vi "Tower_Crane_Jack_Monitor.vi"() -> ()   [LabVIEW 2018]
uses:
  <vilib>/Utility/error.llb/DialogType.ctl
panel:
  out "起升高度（m）":dbl caption="起升高度（cm）" format="%#_3g"
  out "变幅长度（m）":dbl format="%#_3g"
  out "风速（m/s）":dbl format="%.3f"
  out "Y倾斜角度":dbl format="%#_3g"
  out "X倾斜角度":dbl format="%#_3g"
  out "回转角度（°）":dbl format="%#_3g"
  out "回转角度":dbl(knob) scale=0.0..10.0
  out "风速":dbl(knob) scale=0.0..10.0
  out "变幅长度":dbl(knob) scale=0.0..140.0
  out "y轴倾角":dbl(knob) scale=0.0..5.0
  out "x轴倾角":dbl(knob) scale=0.0..5.0
  out "温度计":dbl(slide) caption="顶升高度          (cm)" scale=0.0..180.0
  out "section_connect":picture caption="引进节连接"
  out "rotary_support":picture caption="下回转支座"
  out "stanard_section":picture caption="引进节"
  out "pin_shaft":picture caption="爬爪"
  out "jacking_beam":picture caption="顶升横梁"
  out "new picture":picture caption="Opertion_Guide"
  out "引进滑轮":bool
  out "引进节螺栓4":bool
  out "引进节螺栓3":bool
  out "引进节螺栓2":bool
  out "引进节螺栓1":bool
  out "下回转螺栓4":bool
  out "下回转螺栓3":bool
  out "下回转螺栓2":bool
  out "下回转螺栓1":bool
  out "爬爪右侧":bool
  out "爬爪左侧":bool
  out "横梁右侧":bool
  out "横梁左侧":bool
  in  "停止":bool
  in  "倾角串口号":refnum<visa-resource-name>
  in  "风速串口号":refnum<visa-resource-name>
  in  "回转编码器":refnum<visa-resource-name>
  in  "变幅编码器":refnum<visa-resource-name>
  in  "高度编码器":refnum<visa-resource-name>
  in  "顶升开关":bool
  in  "滚轮直径D":dbl
  out "esp32的IP地址":string
  out "回转圈数":dbl
  out "回转编码器读取缓冲区":string
  out "回转单圈值":dbl
  out "回转编码器错误输出":string
  out "变幅圈数":dbl
  out "小车蝙蝠编码器读取缓冲区":string
  out "变幅单圈值":dbl
  out "回转编码器错误输出1":string
  out "倾角读取缓冲区":string
  out "Wind_Speed_Data":string
  out "风速传感器错误输出":string
  out "操作规范":string
  out "起升圈数":dbl
  out "起升高度编码器读取缓冲区 2":string
  out "起升单圈值":dbl
  out "起升高度编码器数值":dbl
  out "高度编码器错误输出1":string
  out "data out":string
  out "数据输出":string
  out "信息来源的端口":u16
  in  "清空":bool
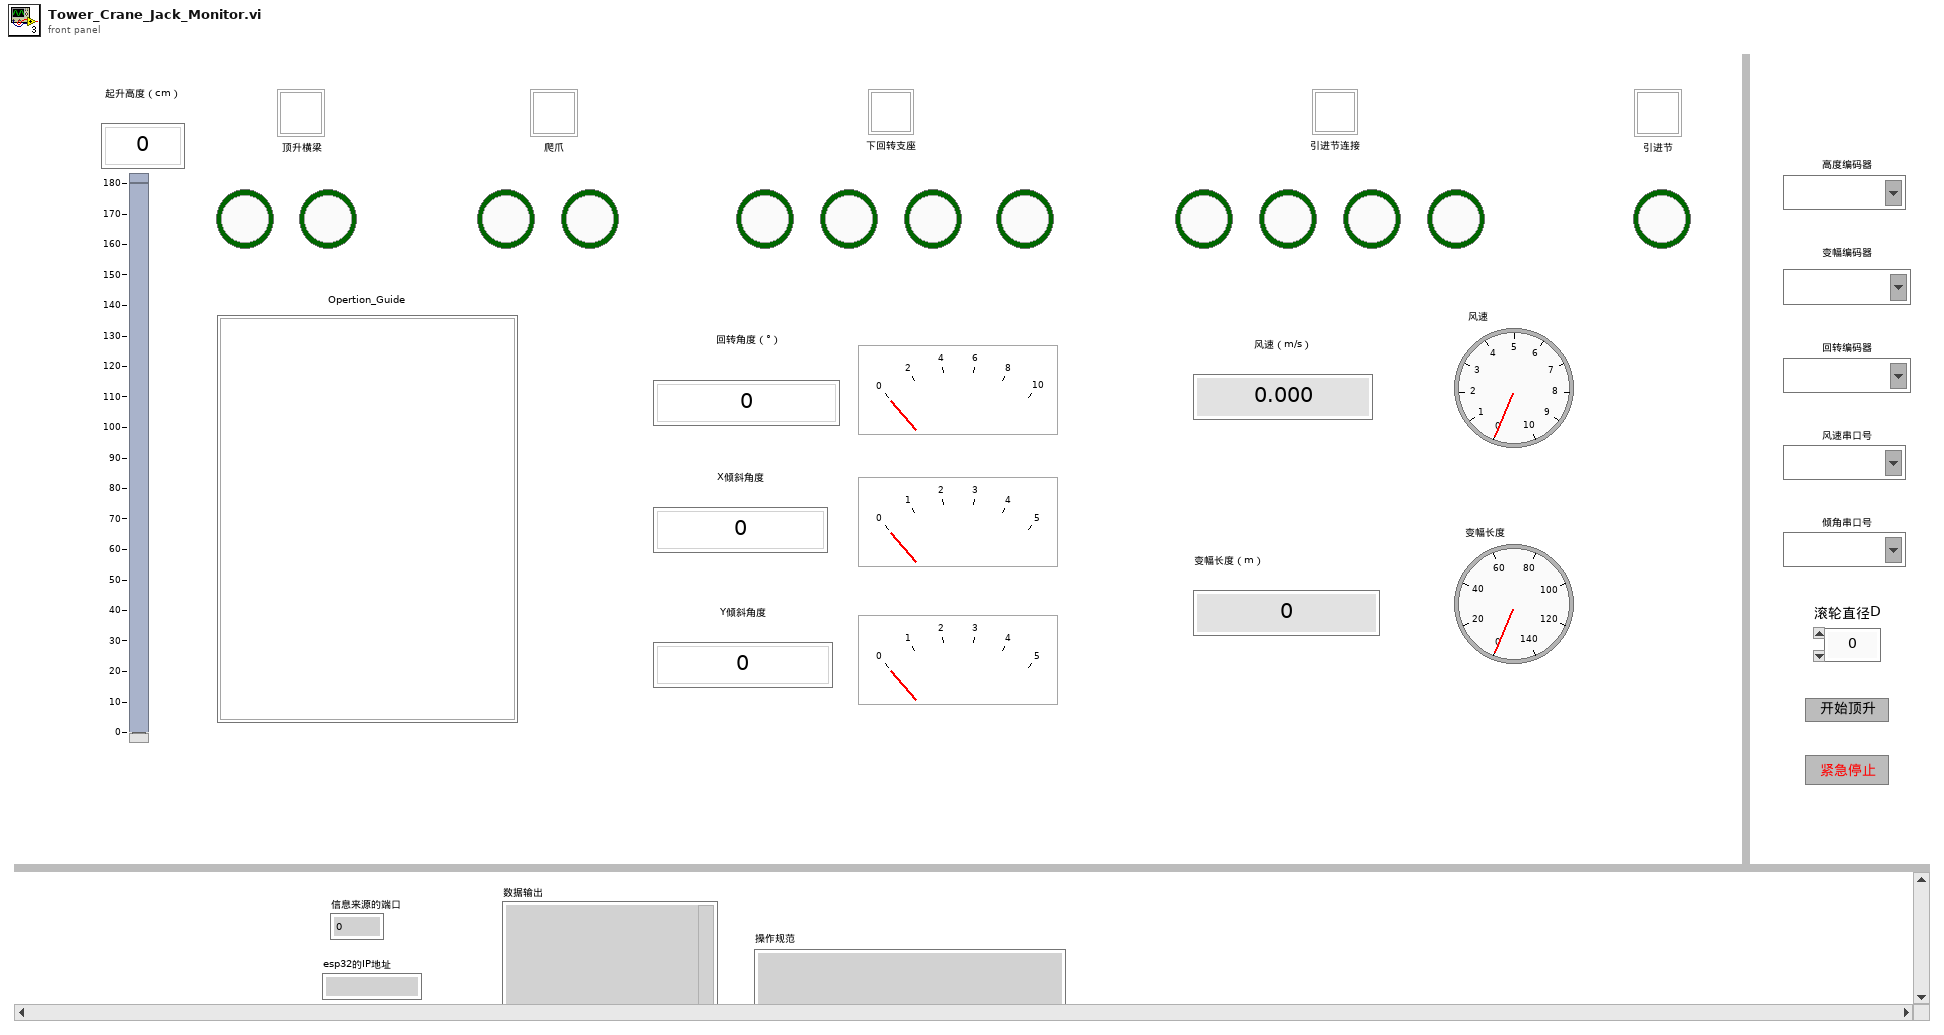
[diagram p1: front panel]
types:
  T1 = typedef "DialogType.ctl" = u16
  T2 = typedef "imagedata.ctl" = cluster{"image type":i32, "image depth":i32, "image":u8[], "mask":u8[], "colors":u32[], "Rectangle":cluster{"left":i16, "top":i16, "right":i16, "bottom":i16}}
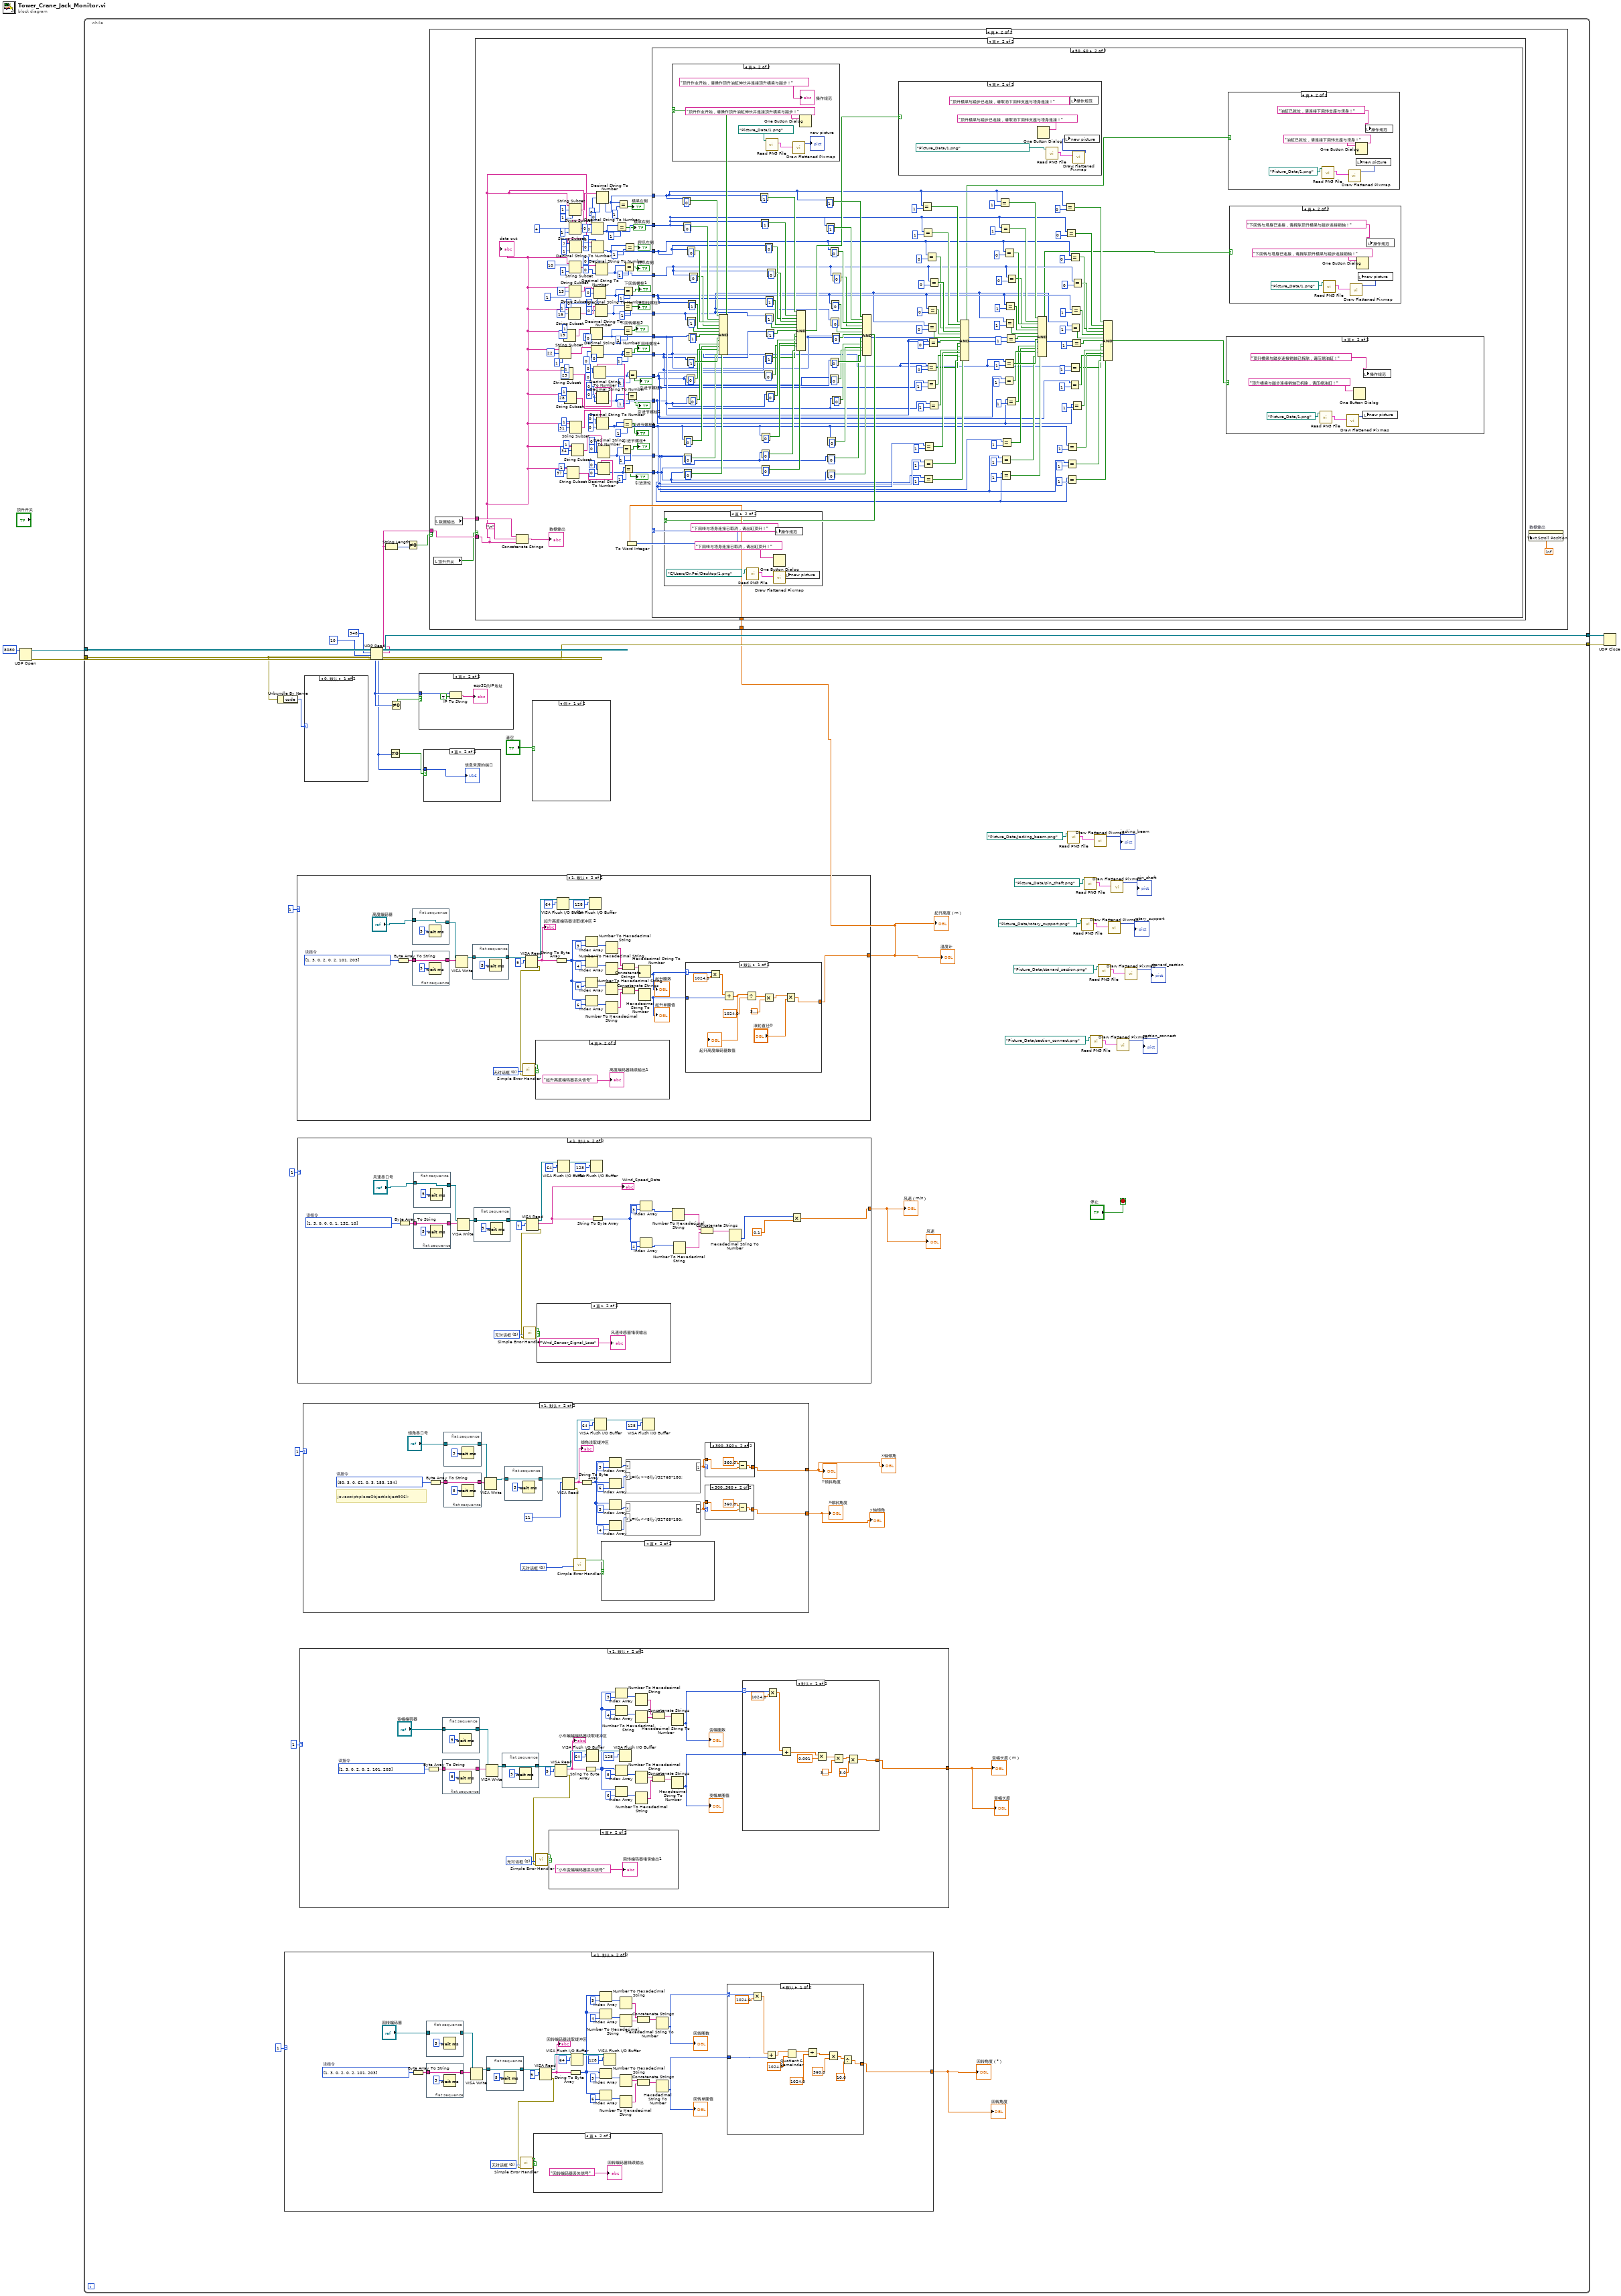
[diagram p0: block diagram]
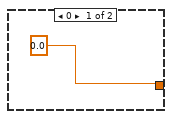
[diagram p2: hidden frame]
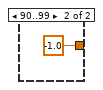
[diagram p4: hidden frame]
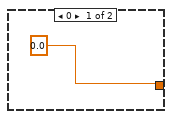
[diagram p5: hidden frame]
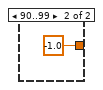
[diagram p7: hidden frame]
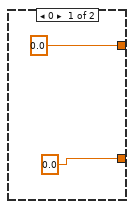
[diagram p8: hidden frame]
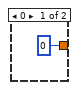
[diagram p12: hidden frame]
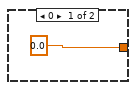
[diagram p14: hidden frame]
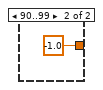
[diagram p16: hidden frame]
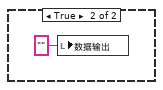
[diagram p17: hidden frame]
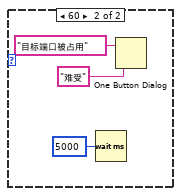
[diagram p18: hidden frame]
diagram:
  n1 = UDP Open(11:u16 8080 ("端口")) -> (port=w5:refnum<k16>, 0:w4:errorcluster)  [unwired: 4 in, 1 out]
  n2 = while {
    tunnel: w5 -> [w47]
    tunnel: w4 -> [w36]
    tunnel: [w46] -> w3
    tunnel: [w43] -> w2
    stop <- "停止" stop-if-true
    n3 = Unbundle By Name(w36) -> ("code"=w35:i32)
    n4 = case shown="1, 默认" 1 {
      tunnel: [0.0 w54] -> w6
      frame 0 {
      }
      frame 1, Default {
        w52 = T1 0 items=["无对话框", "确定信息", "继续或停止信息", "确定信息＋警告", "继续/停止+警告"] ("type of dialog (OK msg:1)")
        w55 = i32[] [1, 3, 0, 2, 0, 2, 101, 203]  # 读指令
        n5 = Byte Array To String(unsigned byte array=w55) -> (string=w72:string)
        n6 = flat-sequence {
          tunnel: "回转编码器" -> [w102]
          tunnel: [w102] -> w49
          frame #0 {
            n7 = Wait (ms)(milliseconds to wait=5) -> ()  [unwired: 1 out]
          }
        }
        n8 = flat-sequence {
          tunnel: [w100] -> w71
          tunnel: w72 -> [w100]
          frame #0 {
            n9 = Wait (ms)(milliseconds to wait=5) -> ()  [unwired: 1 out]
          }
        }
        n10 = VISA Write(VISA resource name=w49, write buffer=w71) -> (VISA resource name out=w63:refnum<visa-resource-name>)  [unwired: 1 in, 2 out]
        n11 = flat-sequence {
          tunnel: [w98] -> w64
          tunnel: w63 -> [w98]
          frame #0 {
            n12 = Wait (ms)(milliseconds to wait=5) -> ()  [unwired: 1 out]
          }
        }
        n13 = VISA Read(VISA resource name=w64, byte count=u32 9 ("字节总数")) -> (VISA resource name out=w80:refnum<visa-resource-name>, read buffer=w70:string, error out=w51:errorcluster)  [unwired: 1 in, 1 out]
        "回转编码器读取缓冲区" <- w70
        n14 = call <vilib>:"Simple Error Handler.vi"("type of dialog (OK msg:1)"=w52, "error in (no error)"=w51) -> ("error?"=w53:bool)  [unwired: 3 in, 4 out]
        n15 = case shown="真" w53 {
          frame False {
          }
          frame True {
            "回转编码器错误输出" <- "回转编码器丢失信号" ("九轴错误输出1")
          }
        }
        n16 = String To Byte Array(string=w70) -> (unsigned byte array=w78:u8[])
        n17 = VISA Flush I/O Buffer(VISA resource name=w80, mask (16)=64) -> (VISA resource name out=w79:refnum<visa-resource-name>)  [unwired: 1 in, 1 out]
        n18 = Index Array ("索引数组")(array=w78, index=3) -> (element=w65:u8)
        n19 = Index Array(array=w78, index=4) -> (element=w69:u8)
        n20 = Index Array ("索引数组")(array=w78, index=5) -> (element=w73:u8)
        n21 = Index Array(array=w78, index=6) -> (element=w77:u8)
        n22 = VISA Flush I/O Buffer(VISA resource name=w79, mask (16)=128) -> ()  [unwired: 1 in, 2 out]
        n23 = Number To Hexadecimal String(2:w65) -> (0:w68:string)  [unwired: 1 in]
        n24 = Number To Hexadecimal String(2:w69) -> (0:w67:string)  [unwired: 1 in]
        n25 = Number To Hexadecimal String(2:w73) -> (0:w76:string)  [unwired: 1 in]
        n26 = Number To Hexadecimal String(2:w77) -> (0:w75:string)  [unwired: 1 in]
        n27 = Concatenate Strings(w68, w67) -> (w66:string)
        n28 = Concatenate Strings(w76, w75) -> (w74:string)
        n29 = Hexadecimal String To Number(string=w66) -> (number=w81:u32)  [unwired: 2 in, 1 out]
        "回转圈数" <- w81
        n30 = Hexadecimal String To Number(string=w74) -> (number=w82:u32)  [unwired: 2 in, 1 out]
        "回转单圈值" <- w82
        n31 = case shown="默认" w81 {
          selector: w81 -> [w94 _]
          tunnel: w82 -> [w93 _]
          tunnel: [w85 -1.0] -> w54
          frame Default {
            n32 = Multiply(x=w94, y=1024.0) -> (x*y=w96:dbl)
            n33 = Add(x=w96, y=w93) -> (x+y=w92:dbl)
            n34 = Quotient & Remainder(x=w92, y=1024.0) -> (x-y*floor(x/y)=w87:dbl)  [unwired: 1 out]
            n35 = Divide(x=w87, y=1024.0) -> (x/y=w89:dbl)
            n36 = Multiply(x=w89, y=360.0) -> (x*y=w86:dbl)
            n37 = Divide(x=w86, y=10.0) -> (x/y=w85:dbl)
          }
          frame 90..99 {
          }
        }
      }
    }
    "回转角度（°）" <- w6
    "回转角度" <- w6
    n38 = case shown="1, 默认" 1 {
      tunnel: [0.0 w244] -> w11
      frame 0 {
      }
      frame 1, Default {
        w242 = T1 0 items=["无对话框", "确定信息", "继续或停止信息", "确定信息＋警告", "继续/停止+警告"] ("type of dialog (OK msg:1)")
        w245 = i32[] [1, 3, 0, 2, 0, 2, 101, 203]  # 读指令
        n39 = Byte Array To String(unsigned byte array=w245) -> (string=w261:string)
        n40 = flat-sequence {
          tunnel: "高度编码器" -> [w290]
          tunnel: [w290] -> w239
          frame #0 {
            n41 = Wait (ms)(milliseconds to wait=5) -> ()  [unwired: 1 out]
          }
        }
        n42 = flat-sequence {
          tunnel: [w288] -> w260
          tunnel: w261 -> [w288]
          frame #0 {
            n43 = Wait (ms)(milliseconds to wait=5) -> ()  [unwired: 1 out]
          }
        }
        n44 = VISA Write(VISA resource name=w239, write buffer=w260) -> (VISA resource name out=w253:refnum<visa-resource-name>)  [unwired: 1 in, 2 out]
        n45 = flat-sequence {
          tunnel: [w286] -> w254
          tunnel: w253 -> [w286]
          frame #0 {
            n46 = Wait (ms)(milliseconds to wait=5) -> ()  [unwired: 1 out]
          }
        }
        n47 = VISA Read(VISA resource name=w254, byte count=u32 9 ("字节总数")) -> (VISA resource name out=w269:refnum<visa-resource-name>, read buffer=w270:string, error out=w241:errorcluster)  [unwired: 1 in, 1 out]
        "起升高度编码器读取缓冲区 2" <- w270
        n48 = call <vilib>:"Simple Error Handler.vi"("type of dialog (OK msg:1)"=w242, "error in (no error)"=w241) -> ("error?"=w243:bool)  [unwired: 3 in, 4 out]
        n49 = case shown="真" w243 {
          frame False {
          }
          frame True {
            "高度编码器错误输出1" <- "起升高度编码器丢失信号" ("九轴错误输出1")
          }
        }
        n50 = String To Byte Array(string=w270) -> (unsigned byte array=w267:u8[])
        n51 = VISA Flush I/O Buffer(VISA resource name=w269, mask (16)=64) -> (VISA resource name out=w268:refnum<visa-resource-name>)  [unwired: 1 in, 1 out]
        n52 = Index Array ("索引数组")(array=w267, index=3) -> (element=w255:u8)
        n53 = Index Array(array=w267, index=4) -> (element=w259:u8)
        n54 = Index Array ("索引数组")(array=w267, index=5) -> (element=w262:u8)
        n55 = Index Array(array=w267, index=6) -> (element=w266:u8)
        n56 = VISA Flush I/O Buffer(VISA resource name=w268, mask (16)=128) -> ()  [unwired: 1 in, 2 out]
        n57 = Number To Hexadecimal String(2:w255) -> (0:w258:string)  [unwired: 1 in]
        n58 = Number To Hexadecimal String(2:w259) -> (0:w257:string)  [unwired: 1 in]
        n59 = Number To Hexadecimal String(2:w262) -> (0:w265:string)  [unwired: 1 in]
        n60 = Number To Hexadecimal String(2:w266) -> (0:w264:string)  [unwired: 1 in]
        n61 = Concatenate Strings(w258, w257) -> (w256:string)
        n62 = Concatenate Strings(w265, w264) -> (w263:string)
        n63 = Hexadecimal String To Number(string=w256) -> (number=w271:u32)  [unwired: 2 in, 1 out]
        "起升圈数" <- w271
        n64 = Hexadecimal String To Number(string=w263) -> (number=w272:u32)  [unwired: 2 in, 1 out]
        "起升单圈值" <- w272
        n65 = case shown="默认" w271 {
          selector: w271 -> [w281 _]
          tunnel: w272 -> [w282 _]
          tunnel: [w274 -1.0] -> w244
          frame Default {
            n66 = Multiply(x=w281, y=1024.0) -> (x*y=w284:dbl)
            n67 = Add(x=w284, y=w282) -> (x+y=w280:dbl)
            "起升高度编码器数值" <- w280
            n68 = Divide(x=w280, y=1024.0) -> (x/y=w278:dbl)
            n69 = Multiply(x=w278, y=3.141592653589793) -> (x*y=w276:dbl)
            n70 = Multiply(x=w276, y="滚轮直径D") -> (x*y=w274:dbl)
          }
          frame 90..99 {
          }
        }
      }
    }
    "起升高度（m）" <- w11
    "温度计" <- w11
    n71 = case shown="1, 默认" 1 {
      tunnel: [u32 0 w205] -> w7
      frame 0 {
      }
      frame 1, Default {
        w219 = T1 0 items=["无对话框", "确定信息", "继续或停止信息", "确定信息＋警告", "继续/停止+警告"] ("type of dialog (OK msg:1)")
        w221 = i32[] [1, 3, 0, 0, 0, 1, 132, 10]  # 读指令
        n72 = Byte Array To String(unsigned byte array=w221) -> (string=w228:string)
        n73 = flat-sequence {
          tunnel: "风速串口号" -> [w236]
          tunnel: [w236] -> w216
          frame #0 {
            n74 = Wait (ms)(milliseconds to wait=5) -> ()  [unwired: 1 out]
          }
        }
        n75 = flat-sequence {
          tunnel: [w234] -> w227
          tunnel: w228 -> [w234]
          frame #0 {
            n76 = Wait (ms)(milliseconds to wait=5) -> ()  [unwired: 1 out]
          }
        }
        n77 = VISA Write(VISA resource name=w216, write buffer=w227) -> (VISA resource name out=w225:refnum<visa-resource-name>)  [unwired: 1 in, 2 out]
        n78 = flat-sequence {
          tunnel: [w232] -> w226
          tunnel: w225 -> [w232]
          frame #0 {
            n79 = Wait (ms)(milliseconds to wait=5) -> ()  [unwired: 1 out]
          }
        }
        n80 = VISA Read(VISA resource name=w226, byte count=u32 7 ("字节总数")) -> (VISA resource name out=w230:refnum<visa-resource-name>, read buffer=w215:string, error out=w218:errorcluster)  [unwired: 1 in, 1 out]
        "Wind_Speed_Data" <- w215
        n81 = call <vilib>:"Simple Error Handler.vi"("type of dialog (OK msg:1)"=w219, "error in (no error)"=w218) -> ("error?"=w220:bool)  [unwired: 3 in, 4 out]
        n82 = case shown="真" w220 {
          frame False {
          }
          frame True {
            "风速传感器错误输出" <- "Wnd_Sensor_Signal_Loss" ("九轴错误输出1")
          }
        }
        n83 = VISA Flush I/O Buffer(VISA resource name=w230, mask (16)=64) -> (VISA resource name out=w229:refnum<visa-resource-name>)  [unwired: 1 in, 1 out]
        n84 = VISA Flush I/O Buffer(VISA resource name=w229, mask (16)=128) -> ()  [unwired: 1 in, 2 out]
        n85 = String To Byte Array(string=w215) -> (unsigned byte array=w214:u8[])
        n86 = Index Array(array=w214, index=3 ("索引")) -> (element=w211:u8)
        n87 = Index Array(array=w214, index=4 ("索引")) -> (element=w210:u8)
        n88 = Number To Hexadecimal String(2:w211) -> (0:w209:string)  [unwired: 1 in]
        n89 = Number To Hexadecimal String(2:w210) -> (0:w208:string)  [unwired: 1 in]
        n90 = Concatenate Strings(w209, w208) -> (w207:string)
        n91 = Hexadecimal String To Number(string=w207) -> (number=w206:u32)  [unwired: 2 in, 1 out]
        n92 = Multiply(x=w206, y=0.1) -> (x*y=w205:dbl)
      }
    }
    "风速" <- w7
    "风速（m/s）" <- w7
    n93 = case shown="1, 默认" 1 {
      tunnel: [0.0 w110] -> w8
      frame 0 {
      }
      frame 1, Default {
        w108 = T1 0 items=["无对话框", "确定信息", "继续或停止信息", "确定信息＋警告", "继续/停止+警告"] ("type of dialog (OK msg:1)")
        w111 = i32[] [1, 3, 0, 2, 0, 2, 101, 203]  # 读指令
        n94 = Byte Array To String(unsigned byte array=w111) -> (string=w128:string)
        n95 = flat-sequence {
          tunnel: "变幅编码器" -> [w156]
          tunnel: [w156] -> w105
          frame #0 {
            n96 = Wait (ms)(milliseconds to wait=5) -> ()  [unwired: 1 out]
          }
        }
        n97 = flat-sequence {
          tunnel: [w154] -> w127
          tunnel: w128 -> [w154]
          frame #0 {
            n98 = Wait (ms)(milliseconds to wait=5) -> ()  [unwired: 1 out]
          }
        }
        n99 = VISA Write(VISA resource name=w105, write buffer=w127) -> (VISA resource name out=w119:refnum<visa-resource-name>)  [unwired: 1 in, 2 out]
        n100 = flat-sequence {
          tunnel: [w152] -> w120
          tunnel: w119 -> [w152]
          frame #0 {
            n101 = Wait (ms)(milliseconds to wait=5) -> ()  [unwired: 1 out]
          }
        }
        n102 = VISA Read(VISA resource name=w120, byte count=u32 9 ("字节总数")) -> (VISA resource name out=w136:refnum<visa-resource-name>, read buffer=w126:string, error out=w107:errorcluster)  [unwired: 1 in, 1 out]
        "小车蝙蝠编码器读取缓冲区" <- w126
        n103 = call <vilib>:"Simple Error Handler.vi"("type of dialog (OK msg:1)"=w108, "error in (no error)"=w107) -> ("error?"=w109:bool)  [unwired: 3 in, 4 out]
        n104 = case shown="真" w109 {
          frame False {
          }
          frame True {
            "回转编码器错误输出1" <- "小车变幅编码器丢失信号" ("九轴错误输出1")
          }
        }
        n105 = String To Byte Array(string=w126) -> (unsigned byte array=w134:u8[])
        n106 = VISA Flush I/O Buffer(VISA resource name=w136, mask (16)=64) -> (VISA resource name out=w135:refnum<visa-resource-name>)  [unwired: 1 in, 1 out]
        n107 = Index Array ("索引数组")(array=w134, index=3) -> (element=w121:u8)
        n108 = Index Array(array=w134, index=4) -> (element=w125:u8)
        n109 = Index Array ("索引数组")(array=w134, index=5) -> (element=w129:u8)
        n110 = Index Array(array=w134, index=6) -> (element=w133:u8)
        n111 = VISA Flush I/O Buffer(VISA resource name=w135, mask (16)=128) -> ()  [unwired: 1 in, 2 out]
        n112 = Number To Hexadecimal String(2:w121) -> (0:w124:string)  [unwired: 1 in]
        n113 = Number To Hexadecimal String(2:w125) -> (0:w123:string)  [unwired: 1 in]
        n114 = Number To Hexadecimal String(2:w129) -> (0:w132:string)  [unwired: 1 in]
        n115 = Number To Hexadecimal String(2:w133) -> (0:w131:string)  [unwired: 1 in]
        n116 = Concatenate Strings(w124, w123) -> (w122:string)
        n117 = Concatenate Strings(w132, w131) -> (w130:string)
        n118 = Hexadecimal String To Number(string=w122) -> (number=w137:u32)  [unwired: 2 in, 1 out]
        "变幅圈数" <- w137
        n119 = Hexadecimal String To Number(string=w130) -> (number=w138:u32)  [unwired: 2 in, 1 out]
        "变幅单圈值" <- w138
        n120 = case shown="默认" w137 {
          selector: w137 -> [w144 _]
          tunnel: w138 -> [w143 _]
          tunnel: [w142 -1.0] -> w110
          frame Default {
            n121 = Multiply(x=w144, y=1024.0) -> (x*y=w149:dbl)
            n122 = Add(x=w149, y=w143) -> (x+y=w150:dbl)
            n123 = Multiply(x=w150, y=0.001) -> (x*y=w147:dbl)
            n124 = Multiply(x=w147, y=3.141592653589793) -> (x*y=w148:dbl)
            n125 = Multiply(x=w148, y=3.0) -> (x*y=w142:dbl)
          }
          frame 90..99 {
          }
        }
      }
    }
    "变幅长度（m）" <- w8
    "变幅长度" <- w8
    n126 = case shown="1, 默认" 1 {
      tunnel: [0.0 w166] -> w10
      tunnel: [0.0 w165] -> w9
      frame 0 {
      }
      frame 1, Default {
        w162 = T1 0 items=["无对话框", "确定信息", "继续或停止信息", "确定信息＋警告", "继续/停止+警告"] ("type of dialog (OK msg:1)")
        w167 = i32[] [80, 3, 0, 61, 0, 3, 153, 134]  # 读指令
        # "javascript:placeObject(object906);"
        n127 = Byte Array To String(unsigned byte array=w167) -> (string=w180:string)
        n128 = flat-sequence {
          tunnel: [w201] -> w161
          tunnel: "倾角串口号" -> [w201]
          frame #0 {
            n129 = Wait (ms)(milliseconds to wait=5) -> ()  [unwired: 1 out]
          }
        }
        n130 = flat-sequence {
          tunnel: [w199] -> w181
          tunnel: w180 -> [w199]
          frame #0 {
            n131 = Wait (ms)(milliseconds to wait=5) -> ()  [unwired: 1 out]
          }
        }
        n132 = VISA Write(VISA resource name=w161, write buffer=w181) -> (VISA resource name out=w176:refnum<visa-resource-name>)  [unwired: 1 in, 2 out]
        n133 = flat-sequence {
          tunnel: w176 -> [w197]
          tunnel: [w197] -> w177
          frame #0 {
            n134 = Wait (ms)(milliseconds to wait=5) -> ()  [unwired: 1 out]
          }
        }
        n135 = VISA Read(VISA resource name=w177, byte count=u32 11 ("字节总数")) -> (VISA resource name out=w185:refnum<visa-resource-name>, read buffer=w175:string, error out=w163:errorcluster)  [unwired: 1 in, 1 out]
        "倾角读取缓冲区" <- w175
        n136 = call <vilib>:"Simple Error Handler.vi"("type of dialog (OK msg:1)"=w162, "error in (no error)"=w163) -> ("error?"=w164:bool)  [unwired: 3 in, 4 out]
        n137 = String To Byte Array(string=w175) -> (unsigned byte array=w186:u8[])
        n138 = VISA Flush I/O Buffer(VISA resource name=w185, mask (16)=64) -> (VISA resource name out=w184:refnum<visa-resource-name>)  [unwired: 1 in, 1 out]
        n139 = case shown="真" w164 {
          frame False {
          }
          frame True {
          }
        }
        n140 = Index Array(array=w186, index=5) -> (element=w183:u8)
        n141 = Index Array(array=w186, index=6) -> (element=w182:u8)
        n142 = Index Array(array=w186, index=3) -> (element=w179:u8)
        n143 = Index Array(array=w186, index=4) -> (element=w178:u8)
        n144 = formula code="z=((x<<8)|y)/32768*180;"("x"=w183, "y"=w182) -> ("z"=w188:dbl)
        n145 = formula code="z=((x<<8)|y)/32768*180;"("x"=w179, "y"=w178) -> ("z"=w187:dbl)
        n146 = VISA Flush I/O Buffer(VISA resource name=w184, mask (16)=128) -> ()  [unwired: 1 in, 2 out]
        n147 = case shown="300..360" w188 {
          tunnel: [w193 w195] -> w166
          tunnel: w188 -> [w193 w194]
          frame Default {
          }
          frame 300..360 {
            n148 = Subtract(x=360.0, y=w194) -> (x-y=w195:dbl)
          }
        }
        n149 = case shown="300..360" w187 {
          tunnel: [w189 w191] -> w165
          tunnel: w187 -> [w189 w190]
          frame Default {
          }
          frame 300..360 {
            n150 = Subtract(x=360.0, y=w190) -> (x-y=w191:dbl)
          }
        }
      }
    }
    "X倾斜角度" <- w9
    "Y倾斜角度" <- w10
    "x轴倾角" <- w10
    "y轴倾角" <- w9
    n151 = case shown="0, 默认" w35 {
      frame 0, Default {
      }
      frame 60 {
        n152 = Wait (ms)(milliseconds to wait=u32 5000 ("等待时间（毫秒）")) -> ()  [unwired: 1 out]
        n153 = One Button Dialog(message="目标端口被占用" ("消息"), button name ("OK")="难受" ("按钮名称（“确定”）")) -> ()  [unwired: 1 out]
      }
    }
    n154 = UDP Read(connection ID=w47, max size (548)=548 ("最大值(548)"), timeout ms (25000)=10 ("超时毫秒(25000)"), 8:w36) -> (data out=w40:string, error out=w46:errorcluster, 3:w43:refnum<k16>, 4:w34:u16, 6:w39:u32)
    n155 = String Length(string=w40) -> (length=w42:i32)
    n156 = Not Equal To 0?(x=w34) -> (x != 0?=w37:bool)
    n157 = Not Equal To 0?(x=w39) -> (x != 0?=w38:bool)
    n158 = Not Equal To 0?(x=w42) -> (x != 0?=w41:bool)
    n159 = case shown="真" w38 {
      tunnel: w39 -> [_ w299]
      frame False {
      }
      frame True {
        n160 = IP To String(1:TRUE ("句点符号？(F)"), 2:w299) -> (0:→"esp32的IP地址":string)
      }
    }
    n161 = case shown="真" w37 {
      tunnel: w34 -> [_ w296]
      frame False {
      }
      frame True {
        "信息来源的端口" <- w296
      }
    }
    n162 = case shown="真" w41 {
      tunnel: w40 -> [_ w303]
      tunnel: w11 -> [_ w301]
      frame False {
      }
      frame True {
        n163 = local read "顶升开关"() -> (w300:bool)
        n164 = local read "数据输出"() -> (w304:string)
        n165 = case shown="真" w300 {
          tunnel: w304 -> [w307 w416]
          tunnel: w303 -> [w306 w391]
          tunnel: w301 -> [_ w394]
          frame False {
            n166 = Concatenate Strings(w307, w306) -> (w305:string)
            n167 = local write "数据输出"(w305) -> ()
          }
          frame True {
            (unwired) 0 ("默认(0 I32)")
            n168 = Concatenate Strings(w416, "\n", w391) -> (→"数据输出":string)
            n169 = String Subset(string=w391, offset (0)=22 ("偏移量(0)"), length (rest)=1 ("长度（剩余）")) -> (substring=w352:string)
            n170 = String Subset(string=w391, offset (0)=25 ("偏移量(0)"), length (rest)=1 ("长度（剩余）")) -> (substring=w351:string)
            n171 = String Subset(string=w391, offset (0)=19 ("偏移量(0)"), length (rest)=1 ("长度（剩余）")) -> (substring=w353:string)
            n172 = String Subset(string=w391, offset (0)=28 ("偏移量(0)"), length (rest)=1 ("长度（剩余）")) -> (substring=w350:string)
            n173 = String Subset(string=w391, offset (0)=37 ("偏移量(0)"), length (rest)=1 ("长度（剩余）")) -> (substring=w347:string)
            n174 = String Subset(string=w391, offset (0)=16 ("偏移量(0)"), length (rest)=1 ("长度（剩余）")) -> (substring=w369:string)
            n175 = String Subset(string=w391, offset (0)=4 ("偏移量(0)"), length (rest)=1 ("长度（剩余）")) -> (substring=w404:string)
            n176 = String Subset(string=w391, offset (0)=13 ("偏移量(0)"), length (rest)=1 ("长度（剩余）")) -> (substring=w370:string)
            n177 = String Subset(string=w391, offset (0)=1 ("偏移量(0)"), length (rest)=1 ("长度（剩余）")) -> (substring=w406:string)
            n178 = String Subset(string=w391, offset (0)=10 ("偏移量(0)"), length (rest)=1 ("长度（剩余）")) -> (substring=w403:string)
            n179 = String Subset(string=w391, offset (0)=31 ("偏移量(0)"), length (rest)=1 ("长度（剩余）")) -> (substring=w349:string)
            n180 = String Subset(string=w391, offset (0)=7 ("偏移量(0)"), length (rest)=1 ("长度（剩余）")) -> (substring=w405:string)
            n181 = String Subset(string=w391, offset (0)=34 ("偏移量(0)"), length (rest)=1 ("长度（剩余）")) -> (substring=w348:string)
            n182 = Decimal String To Number(string=w353, offset=0 ("偏移量"), default (0L)=0 ("默认(0 I32)")) -> (number=w323:i32)  [unwired: 1 out]
            n183 = Decimal String To Number(string=w404, offset=0 ("偏移量"), default (0L)=0 ("默认(0 I32)")) -> (number=w331:i32)  [unwired: 1 out]
            n184 = Decimal String To Number(string=w352, offset=0 ("偏移量"), default (0L)=0 ("默认(0 I32)")) -> (number=w322:i32)  [unwired: 1 out]
            n185 = Decimal String To Number(string=w405, offset=0 ("偏移量"), default (0L)=0 ("默认(0 I32)")) -> (number=w329:i32)  [unwired: 1 out]
            n186 = Decimal String To Number(string=w370, offset=0 ("偏移量"), default (0L)=0 ("默认(0 I32)")) -> (number=w325:i32)  [unwired: 1 out]
            n187 = Decimal String To Number(string=w351, offset=0 ("偏移量")) -> (number=w321:i32)  [unwired: 1 in, 1 out]
            n188 = Decimal String To Number(string=w369, offset=0 ("偏移量"), default (0L)=0 ("默认(0 I32)")) -> (number=w324:i32)  [unwired: 1 out]
            n189 = Decimal String To Number(string=w403, offset=0 ("偏移量"), default (0L)=0 ("默认(0 I32)")) -> (number=w327:i32)  [unwired: 1 out]
            n190 = Decimal String To Number(string=w406, offset=0 ("偏移量"), default (0L)=0 ("默认(0 I32)")) -> (number=w346:i32)  [unwired: 1 out]
            n191 = Decimal String To Number(string=w350, offset=0 ("偏移量"), default (0L)=0 ("默认(0 I32)")) -> (number=w320:i32)  [unwired: 1 out]
            n192 = Decimal String To Number(string=w349, offset=0 ("偏移量"), default (0L)=0 ("默认(0 I32)")) -> (number=w319:i32)  [unwired: 1 out]
            n193 = Decimal String To Number(string=w348, offset=0 ("偏移量"), default (0L)=0 ("默认(0 I32)")) -> (number=w318:i32)  [unwired: 1 out]
            n194 = Decimal String To Number(string=w347, offset=0 ("偏移量"), default (0L)=0 ("默认(0 I32)")) -> (number=w317:i32)  [unwired: 1 out]
            n195 = Equal?(x=w331, y=1) -> (x = y?=→"横梁右侧":bool)
            n196 = Equal?(x=w346, y=1) -> (x = y?=→"横梁左侧":bool)
            n197 = Equal?(x=w318, y=1) -> (x = y?=→"引进节螺栓4":bool)
            n198 = Equal?(x=w319, y=1) -> (x = y?=→"引进节螺栓3":bool)
            n199 = Equal?(x=w324, y=1) -> (x = y?=→"下回转螺栓2":bool)
            n200 = Equal?(x=w323, y=1) -> (x = y?=→"下回转螺栓3":bool)
            n201 = Equal?(x=w322, y=1) -> (x = y?=→"下回转螺栓4":bool)
            n202 = Equal?(x=w325, y=1) -> (x = y?=→"下回转螺栓1":bool)
            n203 = Equal?(x=w317, y=1) -> (x = y?=→"引进滑轮":bool)
            n204 = Equal?(x=w327, y=1) -> (x = y?=→"爬爪右侧":bool)
            n205 = Equal?(x=w329, y=1) -> (x = y?=→"爬爪左侧":bool)
            n206 = To Word Integer(number=w394) -> (16bit integer=w393:i16)
            n207 = Equal?(x=w320, y=1) -> (x = y?=→"引进节螺栓2":bool)
            n208 = Equal?(x=w321, y=1) -> (x = y?=→"引进节螺栓1":bool)
            n209 = case shown="50..60" w393 {
              tunnel: w346 -> [w432 w547 w762 w840 w915 _ w997]
              tunnel: w331 -> [w431 w546 w763 w839 w914 _ w996]
              tunnel: w329 -> [w430 w545 w761 w838 w913 _ w995]
              tunnel: w327 -> [w429 w544 w760 w837 w912 _ w994]
              tunnel: w325 -> [w428 w543 w759 w836 w911 _ w993]
              tunnel: w324 -> [w427 w542 w758 w835 w910 _ w992]
              tunnel: w323 -> [w426 w541 w757 w834 w909 _ w991]
              tunnel: w322 -> [w425 w540 w756 w833 w908 _ w990]
              tunnel: w321 -> [w424 w539 w755 w832 w907 _ w989]
              tunnel: w320 -> [w423 w532 w754 w831 w906 _ w988]
              tunnel: w319 -> [w422 w538 w753 w830 w905 _ w987]
              tunnel: w318 -> [w421 w537 w752 w829 w904 _ w986]
              tunnel: w317 -> [w420 w536 w751 w828 w903 _ w985]
              frame 25..30, Default {
                n210 = Equal?(x=w432, y=0) -> (x = y?=w510:bool)
                n211 = Equal?(x=w431, y=0) -> (x = y?=w509:bool)
                n212 = Equal?(x=w421, y=0) -> (x = y?=w499:bool)
                n213 = Equal?(x=w420, y=0) -> (x = y?=w498:bool)
                n214 = Equal?(x=w422, y=0) -> (x = y?=w500:bool)
                n215 = Equal?(x=w424, y=0) -> (x = y?=w502:bool)
                n216 = Equal?(x=w430, y=1) -> (x = y?=w508:bool)
                n217 = Equal?(x=w425, y=0) -> (x = y?=w503:bool)
                n218 = Equal?(x=w427, y=0) -> (x = y?=w505:bool)
                n219 = Equal?(x=w428, y=0) -> (x = y?=w506:bool)
                n220 = Equal?(x=w426, y=0) -> (x = y?=w504:bool)
                n221 = Equal?(x=w423, y=0) -> (x = y?=w501:bool)
                n222 = Equal?(x=w429, y=1) -> (x = y?=w507:bool)
                n223 = Compound Arithmetic op=AND ("复合运算")(w510, w509, w508, w507, w506, w505, w504, w503, w502, w501, w500, w499, w498) -> (w419:bool)
                n224 = Equal?(x=w432, y=1) -> (x = y?=w485:bool)
                n225 = Equal?(x=w431, y=1) -> (x = y?=w486:bool)
                n226 = Equal?(x=w421, y=0) -> (x = y?=w496:bool)
                n227 = Equal?(x=w420, y=0) -> (x = y?=w497:bool)
                n228 = Equal?(x=w422, y=0) -> (x = y?=w495:bool)
                n229 = Equal?(x=w424, y=0) -> (x = y?=w493:bool)
                n230 = Equal?(x=w430, y=1) -> (x = y?=w487:bool)
                n231 = Equal?(x=w425, y=0) -> (x = y?=w492:bool)
                n232 = Equal?(x=w427, y=0) -> (x = y?=w490:bool)
                n233 = Equal?(x=w428, y=0) -> (x = y?=w489:bool)
                n234 = Equal?(x=w426, y=0) -> (x = y?=w491:bool)
                n235 = Equal?(x=w423, y=0) -> (x = y?=w494:bool)
                n236 = Equal?(x=w429, y=1) -> (x = y?=w488:bool)
                n237 = Compound Arithmetic op=AND ("复合运算")(w485, w486, w487, w488, w489, w490, w491, w492, w493, w494, w495, w496, w497) -> (w418:bool)
                n238 = Equal?(x=w432, y=1) -> (x = y?=w484:bool)
                n239 = Equal?(x=w431, y=1) -> (x = y?=w483:bool)
                n240 = Equal?(x=w421, y=0) -> (x = y?=w473:bool)
                n241 = Equal?(x=w420, y=0) -> (x = y?=w472:bool)
                n242 = Equal?(x=w422, y=0) -> (x = y?=w474:bool)
                n243 = Equal?(x=w424, y=0) -> (x = y?=w476:bool)
                n244 = Equal?(x=w430, y=0) -> (x = y?=w482:bool)
                n245 = Equal?(x=w425, y=0) -> (x = y?=w477:bool)
                n246 = Equal?(x=w427, y=0) -> (x = y?=w479:bool)
                n247 = Equal?(x=w428, y=0) -> (x = y?=w480:bool)
                n248 = Equal?(x=w426, y=0) -> (x = y?=w478:bool)
                n249 = Equal?(x=w423, y=0) -> (x = y?=w475:bool)
                n250 = Equal?(x=w429, y=0) -> (x = y?=w481:bool)
                n251 = Compound Arithmetic op=AND ("复合运算")(w484, w483, w482, w481, w480, w479, w478, w477, w476, w475, w474, w473, w472) -> (w417:bool)
                n252 = case shown="真" w418 {
                  frame False {
                    n253 = call "Empty Picture"() -> ("empty picture"=w512:picture)
                    n254 = local write "new picture"(w512) -> ()
                    n255 = local write "操作规范"("" ("字符串")) -> ()
                  }
                  frame True {
                    n256 = call <vilib>:"Read PNG File.vi"("path to PNG file"=path "Picture_Data/1.png" ("path to JPEG file")) -> ("image data"=w517:T2)  [unwired: 8 in, 2 out]
                    n257 = call <vilib>:"Draw Flattened Pixmap.vi"("image data"=w517) -> ("new picture"=w513:picture)  [unwired: 8 in]
                    n258 = One Button Dialog(message="顶升横梁与踏步连接销轴已连接，请掀起爬爪！" ("消息")) -> ()  [unwired: 1 in, 1 out]
                    n259 = local write "操作规范"("顶升横梁与踏步连接销轴已连接，请掀起爬爪！" ("字符串")) -> ()
                    n260 = local write "new picture"(w513) -> ()
                  }
                }
                n261 = case shown="真" w419 {
                  frame False {
                    n262 = call "Empty Picture"() -> ("empty picture"=w525:picture)
                    n263 = local write "new picture"(w525) -> ()
                    n264 = local write "操作规范"("" ("字符串")) -> ()
                  }
                  frame True {
                    n265 = call <vilib>:"Read PNG File.vi"("path to PNG file"=path "Picture_Data/1.png" ("path to JPEG file")) -> ("image data"=w531:T2)  [unwired: 8 in, 2 out]
                    n266 = call <vilib>:"Draw Flattened Pixmap.vi"("image data"=w531) -> ("new picture"=w527:picture)  [unwired: 8 in]
                    n267 = One Button Dialog(message="油缸压缩完毕，请连接顶升横梁与踏步连接销轴！" ("消息")) -> ()  [unwired: 1 in, 1 out]
                    n268 = local write "操作规范"("油缸压缩完毕，请连接顶升横梁与踏步连接销轴！" ("字符串")) -> ()
                    n269 = local write "new picture"(w527) -> ()
                  }
                }
                n270 = case shown="真" w417 {
                  frame False {
                    n271 = call "Empty Picture"() -> ("empty picture"=w518:picture)
                    n272 = local write "new picture"(w518) -> ()
                    n273 = local write "操作规范"("" ("字符串")) -> ()
                  }
                  frame True {
                    n274 = call <vilib>:"Read PNG File.vi"("path to PNG file"=path "Picture_Data/1.png" ("path to JPEG file")) -> ("image data"=w524:T2)  [unwired: 8 in, 2 out]
                    n275 = call <vilib>:"Draw Flattened Pixmap.vi"("image data"=w524) -> ("new picture"=w521:picture)  [unwired: 8 in]
                    n276 = local write "操作规范"("爬爪已掀起，请出缸顶升至容纳引进节！" ("字符串")) -> ()
                    n277 = One Button Dialog(message="爬爪已掀起，请出缸顶升至容纳引进节！" ("消息")) -> ()  [unwired: 1 in, 1 out]
                    n278 = local write "new picture"(w521) -> ()
                  }
                }
              }
              frame 50..60 {
                n279 = Equal?(x=w547, y=0) -> (x = y?=w706:bool)
                n280 = Equal?(x=w546, y=0) -> (x = y?=w705:bool)
                n281 = Equal?(x=w537, y=0) -> (x = y?=w695:bool)
                n282 = Equal?(x=w536, y=0) -> (x = y?=w694:bool)
                n283 = Equal?(x=w538, y=0) -> (x = y?=w696:bool)
                n284 = Equal?(x=w539, y=0) -> (x = y?=w698:bool)
                n285 = Equal?(x=w545, y=0) -> (x = y?=w704:bool)
                n286 = Equal?(x=w540, y=1) -> (x = y?=w699:bool)
                n287 = Equal?(x=w542, y=1) -> (x = y?=w701:bool)
                n288 = Equal?(x=w543, y=1) -> (x = y?=w702:bool)
                n289 = Equal?(x=w541, y=1) -> (x = y?=w700:bool)
                n290 = Equal?(x=w532, y=0) -> (x = y?=w697:bool)
                n291 = Equal?(x=w544, y=0) -> (x = y?=w703:bool)
                n292 = Compound Arithmetic op=AND ("复合运算")(w706, w705, w704, w703, w702, w701, w700, w699, w698, w697, w696, w695, w694) -> (w628:bool)
                n293 = case shown="真" w628 {
                  frame False {
                    n294 = call "Empty Picture"() -> ("empty picture"=w743:picture)
                    n295 = local write "new picture"(w743) -> ()
                    n296 = local write "操作规范"("" ("字符串")) -> ()
                  }
                  frame True {
                    n297 = call <vilib>:"Read PNG File.vi"("path to PNG file"=path "Picture_Data/1.png" ("path to JPEG file")) -> ("image data"=w747:T2)  [unwired: 8 in, 2 out]
                    n298 = call <vilib>:"Draw Flattened Pixmap.vi"("image data"=w747) -> ("new picture"=→"new picture":picture)  [unwired: 8 in]
                    n299 = One Button Dialog(message="顶升作业开始，请操作顶升油缸伸长并连接顶升横梁与踏步！" ("消息")) -> ()  [unwired: 1 in, 1 out]
                    "操作规范" <- "顶升作业开始，请操作顶升油缸伸长并连接顶升横梁与踏步！" ("字符串")
                  }
                }
                n300 = Equal?(x=w547, y=1) -> (x = y?=w681:bool)
                n301 = Equal?(x=w546, y=1) -> (x = y?=w682:bool)
                n302 = Equal?(x=w537, y=0) -> (x = y?=w692:bool)
                n303 = Equal?(x=w536, y=0) -> (x = y?=w693:bool)
                n304 = Equal?(x=w538, y=0) -> (x = y?=w691:bool)
                n305 = Equal?(x=w539, y=0) -> (x = y?=w689:bool)
                n306 = Equal?(x=w545, y=0) -> (x = y?=w683:bool)
                n307 = Equal?(x=w540, y=1) -> (x = y?=w688:bool)
                n308 = Equal?(x=w542, y=1) -> (x = y?=w686:bool)
                n309 = Equal?(x=w543, y=1) -> (x = y?=w685:bool)
                n310 = Equal?(x=w541, y=1) -> (x = y?=w687:bool)
                n311 = Equal?(x=w532, y=0) -> (x = y?=w690:bool)
                n312 = Equal?(x=w544, y=0) -> (x = y?=w684:bool)
                n313 = Compound Arithmetic op=AND ("复合运算")(w681, w682, w683, w684, w685, w686, w687, w688, w689, w690, w691, w692, w693) -> (w548:bool)
                n314 = Equal?(x=w547, y=1) -> (x = y?=w680:bool)
                n315 = Equal?(x=w546, y=1) -> (x = y?=w679:bool)
                n316 = Equal?(x=w537, y=0) -> (x = y?=w669:bool)
                n317 = Equal?(x=w536, y=0) -> (x = y?=w668:bool)
                n318 = Equal?(x=w538, y=0) -> (x = y?=w670:bool)
                n319 = Equal?(x=w539, y=0) -> (x = y?=w672:bool)
                n320 = Equal?(x=w545, y=0) -> (x = y?=w678:bool)
                n321 = Equal?(x=w540, y=0) -> (x = y?=w673:bool)
                n322 = Equal?(x=w542, y=0) -> (x = y?=w675:bool)
                n323 = Equal?(x=w543, y=0) -> (x = y?=w676:bool)
                n324 = Equal?(x=w541, y=0) -> (x = y?=w674:bool)
                n325 = Equal?(x=w532, y=0) -> (x = y?=w671:bool)
                n326 = Equal?(x=w544, y=0) -> (x = y?=w677:bool)
                n327 = Compound Arithmetic op=AND ("复合运算")(w680, w679, w678, w677, w676, w675, w674, w673, w672, w671, w670, w669, w668) -> (w627:bool)
                n328 = case shown="真" w627 {
                  frame False {
                    n329 = call "Empty Picture"() -> ("empty picture"=w729:picture)
                    n330 = local write "new picture"(w729) -> ()
                    n331 = local write "操作规范"("" ("字符串")) -> ()
                  }
                  frame True {
                    n332 = call <vilib>:"Read PNG File.vi"("path to PNG file"=path "C:/Users/Dr.Pei/Desktop/1.png" ("path to JPEG file")) -> ("image data"=w733:T2)  [unwired: 8 in, 2 out]
                    n333 = One Button Dialog(message="下回转与塔身连接已取消，请出缸顶升！" ("消息")) -> ()  [unwired: 1 in, 1 out]
                    n334 = call <vilib>:"Draw Flattened Pixmap.vi"("image data"=w733) -> ("new picture"=w732:picture)  [unwired: 8 in]
                    n335 = local write "操作规范"("下回转与塔身连接已取消，请出缸顶升！" ("字符串")) -> ()
                    n336 = local write "new picture"(w732) -> ()
                  }
                }
                n337 = case shown="真" w548 {
                  frame False {
                    n338 = call "Empty Picture"() -> ("empty picture"=w736:picture)
                    n339 = local write "操作规范"("" ("字符串")) -> ()
                    n340 = local write "new picture"(w736) -> ()
                  }
                  frame True {
                    n341 = One Button Dialog(message="顶升横梁与踏步已连接，请取消下回转支座与塔身连接！" ("消息")) -> ()  [unwired: 1 in, 1 out]
                    n342 = call <vilib>:"Read PNG File.vi"("path to PNG file"=path "Picture_Data/1.png" ("path to JPEG file")) -> ("image data"=w740:T2)  [unwired: 8 in, 2 out]
                    n343 = local write "操作规范"("顶升横梁与踏步已连接，请取消下回转支座与塔身连接！" ("字符串")) -> ()
                    n344 = call <vilib>:"Draw Flattened Pixmap.vi"("image data"=w740) -> ("new picture"=w739:picture)  [unwired: 8 in]
                    n345 = local write "new picture"(w739) -> ()
                  }
                }
                n346 = Equal?(x=w547, y=1) -> (x = y?=w549:bool)
                n347 = Equal?(x=w546, y=1) -> (x = y?=w550:bool)
                n348 = Equal?(x=w537, y=1) -> (x = y?=w560:bool)
                n349 = Equal?(x=w536, y=1) -> (x = y?=w561:bool)
                n350 = Equal?(x=w538, y=1) -> (x = y?=w559:bool)
                n351 = Equal?(x=w539, y=1) -> (x = y?=w557:bool)
                n352 = Equal?(x=w545, y=0) -> (x = y?=w551:bool)
                n353 = Equal?(x=w540, y=0) -> (x = y?=w556:bool)
                n354 = Equal?(x=w542, y=0) -> (x = y?=w554:bool)
                n355 = Equal?(x=w543, y=0) -> (x = y?=w553:bool)
                n356 = Equal?(x=w541, y=0) -> (x = y?=w555:bool)
                n357 = Equal?(x=w532, y=1) -> (x = y?=w558:bool)
                n358 = Equal?(x=w544, y=0) -> (x = y?=w552:bool)
                n359 = Compound Arithmetic op=AND ("复合运算")(w549, w550, w551, w552, w553, w554, w555, w556, w557, w558, w559, w560, w561) -> (w535:bool)
                n360 = Equal?(x=w547, y=1) -> (x = y?=w574:bool)
                n361 = Equal?(x=w546, y=1) -> (x = y?=w573:bool)
                n362 = Equal?(x=w537, y=1) -> (x = y?=w563:bool)
                n363 = Equal?(x=w536, y=1) -> (x = y?=w562:bool)
                n364 = Equal?(x=w538, y=1) -> (x = y?=w564:bool)
                n365 = Equal?(x=w539, y=1) -> (x = y?=w566:bool)
                n366 = Equal?(x=w545, y=0) -> (x = y?=w572:bool)
                n367 = Equal?(x=w540, y=1) -> (x = y?=w567:bool)
                n368 = Equal?(x=w542, y=1) -> (x = y?=w569:bool)
                n369 = Equal?(x=w543, y=1) -> (x = y?=w570:bool)
                n370 = Equal?(x=w541, y=1) -> (x = y?=w568:bool)
                n371 = Equal?(x=w532, y=1) -> (x = y?=w565:bool)
                n372 = Equal?(x=w544, y=0) -> (x = y?=w571:bool)
                n373 = Compound Arithmetic op=AND ("复合运算")(w574, w573, w572, w571, w570, w569, w568, w567, w566, w565, w564, w563, w562) -> (w534:bool)
                n374 = Equal?(x=w547, y=0) -> (x = y?=w575:bool)
                n375 = Equal?(x=w546, y=0) -> (x = y?=w576:bool)
                n376 = Equal?(x=w537, y=1) -> (x = y?=w586:bool)
                n377 = Equal?(x=w536, y=1) -> (x = y?=w587:bool)
                n378 = Equal?(x=w538, y=1) -> (x = y?=w585:bool)
                n379 = Equal?(x=w539, y=1) -> (x = y?=w583:bool)
                n380 = Equal?(x=w545, y=0) -> (x = y?=w577:bool)
                n381 = Equal?(x=w540, y=1) -> (x = y?=w582:bool)
                n382 = Equal?(x=w542, y=1) -> (x = y?=w580:bool)
                n383 = Equal?(x=w543, y=1) -> (x = y?=w579:bool)
                n384 = Equal?(x=w541, y=1) -> (x = y?=w581:bool)
                n385 = Equal?(x=w532, y=1) -> (x = y?=w584:bool)
                n386 = Equal?(x=w544, y=0) -> (x = y?=w578:bool)
                n387 = Compound Arithmetic op=AND ("复合运算")(w575, w576, w577, w578, w579, w580, w581, w582, w583, w584, w585, w586, w587) -> (w533:bool)
                n388 = case shown="真" w533 {
                  frame False {
                    n389 = call "Empty Picture"() -> ("empty picture"=w707:picture)
                    n390 = local write "new picture"(w707) -> ()
                    n391 = local write "操作规范"("" ("字符串")) -> ()
                  }
                  frame True {
                    n392 = call <vilib>:"Read PNG File.vi"("path to PNG file"=path "Picture_Data/1.png" ("path to JPEG file")) -> ("image data"=w713:T2)  [unwired: 8 in, 2 out]
                    n393 = call <vilib>:"Draw Flattened Pixmap.vi"("image data"=w713) -> ("new picture"=w709:picture)  [unwired: 8 in]
                    n394 = One Button Dialog(message="顶升横梁与踏步连接销轴已拆除，请压缩油缸！" ("消息")) -> ()  [unwired: 1 in, 1 out]
                    n395 = local write "new picture"(w709) -> ()
                    n396 = local write "操作规范"("顶升横梁与踏步连接销轴已拆除，请压缩油缸！" ("字符串")) -> ()
                  }
                }
                n397 = case shown="真" w535 {
                  frame False {
                    n398 = call "Empty Picture"() -> ("empty picture"=w721:picture)
                    n399 = local write "new picture"(w721) -> ()
                    n400 = local write "操作规范"("" ("字符串")) -> ()
                  }
                  frame True {
                    n401 = call <vilib>:"Read PNG File.vi"("path to PNG file"=path "Picture_Data/1.png" ("path to JPEG file")) -> ("image data"=w727:T2)  [unwired: 8 in, 2 out]
                    n402 = call <vilib>:"Draw Flattened Pixmap.vi"("image data"=w727) -> ("new picture"=w723:picture)  [unwired: 8 in]
                    n403 = One Button Dialog(message="油缸已就位，请连接下回转支座与塔身！" ("消息")) -> ()  [unwired: 1 in, 1 out]
                    n404 = local write "new picture"(w723) -> ()
                    n405 = local write "操作规范"("油缸已就位，请连接下回转支座与塔身！" ("字符串")) -> ()
                  }
                }
                n406 = case shown="真" w534 {
                  frame False {
                    n407 = call "Empty Picture"() -> ("empty picture"=w714:picture)
                    n408 = local write "new picture"(w714) -> ()
                    n409 = local write "操作规范"("" ("字符串")) -> ()
                  }
                  frame True {
                    n410 = call <vilib>:"Read PNG File.vi"("path to PNG file"=path "Picture_Data/1.png" ("path to JPEG file")) -> ("image data"=w720:T2)  [unwired: 8 in, 2 out]
                    n411 = call <vilib>:"Draw Flattened Pixmap.vi"("image data"=w720) -> ("new picture"=w716:picture)  [unwired: 8 in]
                    n412 = One Button Dialog(message="下回转与塔身已连接，请拆除顶升横梁与踏步连接销轴！" ("消息")) -> ()  [unwired: 1 in, 1 out]
                    n413 = local write "new picture"(w716) -> ()
                    n414 = local write "操作规范"("下回转与塔身已连接，请拆除顶升横梁与踏步连接销轴！" ("字符串")) -> ()
                  }
                }
              }
              frame 158..168 {
                n415 = Equal?(x=w762, y=1) -> (x = y?=w815:bool)
                n416 = Equal?(x=w763, y=1) -> (x = y?=w814:bool)
                n417 = Equal?(x=w752, y=0) -> (x = y?=w804:bool)
                n418 = Equal?(x=w751, y=0) -> (x = y?=w803:bool)
                n419 = Equal?(x=w753, y=0) -> (x = y?=w805:bool)
                n420 = Equal?(x=w755, y=0) -> (x = y?=w807:bool)
                n421 = Equal?(x=w761, y=0) -> (x = y?=w813:bool)
                n422 = Equal?(x=w756, y=0) -> (x = y?=w808:bool)
                n423 = Equal?(x=w758, y=0) -> (x = y?=w810:bool)
                n424 = Equal?(x=w759, y=0) -> (x = y?=w811:bool)
                n425 = Equal?(x=w757, y=0) -> (x = y?=w809:bool)
                n426 = Equal?(x=w754, y=0) -> (x = y?=w806:bool)
                n427 = Equal?(x=w760, y=0) -> (x = y?=w812:bool)
                n428 = Compound Arithmetic op=AND ("复合运算")(w815, w814, w813, w812, w811, w810, w809, w808, w807, w806, w805, w804, w803) -> (w750:bool)
                n429 = Equal?(x=w762, y=1) -> (x = y?=w790:bool)
                n430 = Equal?(x=w763, y=1) -> (x = y?=w791:bool)
                n431 = Equal?(x=w752, y=0) -> (x = y?=w801:bool)
                n432 = Equal?(x=w751, y=0) -> (x = y?=w802:bool)
                n433 = Equal?(x=w753, y=0) -> (x = y?=w800:bool)
                n434 = Equal?(x=w755, y=0) -> (x = y?=w798:bool)
                n435 = Equal?(x=w761, y=1) -> (x = y?=w792:bool)
                n436 = Equal?(x=w756, y=0) -> (x = y?=w797:bool)
                n437 = Equal?(x=w758, y=0) -> (x = y?=w795:bool)
                n438 = Equal?(x=w759, y=0) -> (x = y?=w794:bool)
                n439 = Equal?(x=w757, y=0) -> (x = y?=w796:bool)
                n440 = Equal?(x=w754, y=0) -> (x = y?=w799:bool)
                n441 = Equal?(x=w760, y=1) -> (x = y?=w793:bool)
                n442 = Compound Arithmetic op=AND ("复合运算")(w790, w791, w792, w793, w794, w795, w796, w797, w798, w799, w800, w801, w802) -> (w749:bool)
                n443 = case shown="真" w750 {
                  frame False {
                    (unwired) "" ("字符串")
                    n444 = call "Empty Picture"() -> ()  [unwired: 1 out]
                  }
                  frame True {
                    n445 = call <vilib>:"Read PNG File.vi"("path to PNG file"=path "Picture_Data/1.png" ("path to JPEG file")) -> ("image data"=w825:T2)  [unwired: 8 in, 2 out]
                    n446 = local write "操作规范"("顶升油缸已到位，请压下爬爪！" ("字符串")) -> ()
                    n447 = call <vilib>:"Draw Flattened Pixmap.vi"("image data"=w825) -> ("new picture"=w821:picture)  [unwired: 8 in]
                    n448 = One Button Dialog(message="顶升油缸已到位，请压下爬爪！" ("消息")) -> ()  [unwired: 1 in, 1 out]
                    n449 = local write "new picture"(w821) -> ()
                  }
                }
                n450 = case shown="真" w749 {
                  frame False {
                    (unwired) "" ("字符串")
                    n451 = call "Empty Picture"() -> ()  [unwired: 1 out]
                  }
                  frame True {
                    n452 = call <vilib>:"Read PNG File.vi"("path to PNG file"=path "Picture_Data/1.png" ("path to JPEG file")) -> ("image data"=w820:T2)  [unwired: 8 in, 2 out]
                    n453 = local write "操作规范"("爬爪已就位，请压缩油缸！" ("字符串")) -> ()
                    n454 = call <vilib>:"Draw Flattened Pixmap.vi"("image data"=w820) -> ("new picture"=w816:picture)  [unwired: 8 in]
                    n455 = One Button Dialog(message="爬爪已就位，请压缩油缸！" ("消息")) -> ()  [unwired: 1 in, 1 out]
                    n456 = local write "new picture"(w816) -> ()
                  }
                }
              }
              frame 150..155 {
                n457 = Equal?(x=w840, y=1) -> (x = y?=w892:bool)
                n458 = Equal?(x=w839, y=1) -> (x = y?=w891:bool)
                n459 = Equal?(x=w829, y=0) -> (x = y?=w881:bool)
                n460 = Equal?(x=w828, y=0) -> (x = y?=w880:bool)
                n461 = Equal?(x=w830, y=0) -> (x = y?=w882:bool)
                n462 = Equal?(x=w832, y=0) -> (x = y?=w884:bool)
                n463 = Equal?(x=w838, y=1) -> (x = y?=w890:bool)
                n464 = Equal?(x=w833, y=0) -> (x = y?=w885:bool)
                n465 = Equal?(x=w835, y=0) -> (x = y?=w887:bool)
                n466 = Equal?(x=w836, y=0) -> (x = y?=w888:bool)
                n467 = Equal?(x=w834, y=0) -> (x = y?=w886:bool)
                n468 = Equal?(x=w831, y=0) -> (x = y?=w883:bool)
                n469 = Equal?(x=w837, y=1) -> (x = y?=w889:bool)
                n470 = Compound Arithmetic op=AND ("复合运算")(w892, w891, w890, w889, w888, w887, w886, w885, w884, w883, w882, w881, w880) -> (w827:bool)
                n471 = Equal?(x=w840, y=0) -> (x = y?=w867:bool)
                n472 = Equal?(x=w839, y=0) -> (x = y?=w868:bool)
                n473 = Equal?(x=w829, y=0) -> (x = y?=w878:bool)
                n474 = Equal?(x=w828, y=0) -> (x = y?=w879:bool)
                n475 = Equal?(x=w830, y=0) -> (x = y?=w877:bool)
                n476 = Equal?(x=w832, y=0) -> (x = y?=w875:bool)
                n477 = Equal?(x=w838, y=1) -> (x = y?=w869:bool)
                n478 = Equal?(x=w833, y=0) -> (x = y?=w874:bool)
                n479 = Equal?(x=w835, y=0) -> (x = y?=w872:bool)
                n480 = Equal?(x=w836, y=0) -> (x = y?=w871:bool)
                n481 = Equal?(x=w834, y=0) -> (x = y?=w873:bool)
                n482 = Equal?(x=w831, y=0) -> (x = y?=w876:bool)
                n483 = Equal?(x=w837, y=1) -> (x = y?=w870:bool)
                n484 = Compound Arithmetic op=AND ("复合运算")(w867, w868, w869, w870, w871, w872, w873, w874, w875, w876, w877, w878, w879) -> (w826:bool)
                n485 = case shown="真" w826 {
                  frame False {
                    (unwired) "" ("字符串")
                    n486 = call "Empty Picture"() -> ()  [unwired: 1 out]
                  }
                  frame True {
                    n487 = call <vilib>:"Read PNG File.vi"("path to PNG file"=path "Picture_Data/1.png" ("path to JPEG file")) -> ("image data"=w897:T2)  [unwired: 8 in, 2 out]
                    n488 = call <vilib>:"Draw Flattened Pixmap.vi"("image data"=w897) -> ("new picture"=w893:picture)  [unwired: 8 in]
                    n489 = One Button Dialog(message="顶升横梁与踏步连接销轴已拆除，请压缩油缸！" ("消息")) -> ()  [unwired: 1 in, 1 out]
                    n490 = local write "操作规范"("顶升横梁与踏步连接销轴已拆除，请压缩油缸！" ("字符串")) -> ()
                    n491 = local write "new picture"(w893) -> ()
                  }
                }
                n492 = case shown="真" w827 {
                  frame False {
                    (unwired) "" ("字符串")
                    n493 = call "Empty Picture"() -> ()  [unwired: 1 out]
                  }
                  frame True {
                    n494 = call <vilib>:"Read PNG File.vi"("path to PNG file"=path "Picture_Data/1.png" ("path to JPEG file")) -> ("image data"=w902:T2)  [unwired: 8 in, 2 out]
                    n495 = call <vilib>:"Draw Flattened Pixmap.vi"("image data"=w902) -> ("new picture"=w898:picture)  [unwired: 8 in]
                    n496 = One Button Dialog(message="油缸已回缩就位，请拆除顶升横梁与踏步连接销轴！" ("消息")) -> ()  [unwired: 1 in, 1 out]
                    n497 = local write "操作规范"("油缸已回缩就位，请拆除顶升横梁与踏步连接销轴！" ("字符串")) -> ()
                    n498 = local write "new picture"(w898) -> ()
                  }
                }
              }
              frame 120..130 {
                n499 = Equal?(x=w915, y=1) -> (x = y?=w969:bool)
                n500 = Equal?(x=w914, y=1) -> (x = y?=w968:bool)
                n501 = Equal?(x=w904, y=0) -> (x = y?=w958:bool)
                n502 = Equal?(x=w903, y=0) -> (x = y?=w957:bool)
                n503 = Equal?(x=w905, y=0) -> (x = y?=w959:bool)
                n504 = Equal?(x=w907, y=0) -> (x = y?=w961:bool)
                n505 = Equal?(x=w913, y=0) -> (x = y?=w967:bool)
                n506 = Equal?(x=w908, y=0) -> (x = y?=w962:bool)
                n507 = Equal?(x=w910, y=0) -> (x = y?=w964:bool)
                n508 = Equal?(x=w911, y=0) -> (x = y?=w965:bool)
                n509 = Equal?(x=w909, y=0) -> (x = y?=w963:bool)
                n510 = Equal?(x=w906, y=0) -> (x = y?=w960:bool)
                n511 = Equal?(x=w912, y=0) -> (x = y?=w966:bool)
                n512 = Compound Arithmetic op=AND ("复合运算")(w969, w968, w967, w966, w965, w964, w963, w962, w961, w960, w959, w958, w957) -> (w917:bool)
                n513 = Equal?(x=w915, y=1) -> (x = y?=w944:bool)
                n514 = Equal?(x=w914, y=1) -> (x = y?=w945:bool)
                n515 = Equal?(x=w904, y=0) -> (x = y?=w955:bool)
                n516 = Equal?(x=w903, y=1) -> (x = y?=w956:bool)
                n517 = Equal?(x=w905, y=0) -> (x = y?=w954:bool)
                n518 = Equal?(x=w907, y=0) -> (x = y?=w952:bool)
                n519 = Equal?(x=w913, y=0) -> (x = y?=w946:bool)
                n520 = Equal?(x=w908, y=0) -> (x = y?=w951:bool)
                n521 = Equal?(x=w910, y=0) -> (x = y?=w949:bool)
                n522 = Equal?(x=w911, y=0) -> (x = y?=w948:bool)
                n523 = Equal?(x=w909, y=0) -> (x = y?=w950:bool)
                n524 = Equal?(x=w906, y=0) -> (x = y?=w953:bool)
                n525 = Equal?(x=w912, y=0) -> (x = y?=w947:bool)
                n526 = Compound Arithmetic op=AND ("复合运算")(w944, w945, w946, w947, w948, w949, w950, w951, w952, w953, w954, w955, w956) -> (w916:bool)
                n527 = case shown="真" w917 {
                  frame False {
                    n528 = call "Empty Picture"() -> ("empty picture"=w978:picture)
                    n529 = local write "操作规范"("" ("字符串")) -> ()
                    n530 = local write "new picture"(w978) -> ()
                  }
                  frame True {
                    n531 = call <vilib>:"Read PNG File.vi"("path to PNG file"=path "Picture_Data/1.png" ("path to JPEG file")) -> ("image data"=w983:T2)  [unwired: 8 in, 2 out]
                    n532 = call <vilib>:"Draw Flattened Pixmap.vi"("image data"=w983) -> ("new picture"=w979:picture)  [unwired: 8 in]
                    n533 = One Button Dialog(message="顶升油缸已就位，请引进新标准节！" ("消息")) -> ()  [unwired: 1 in, 1 out]
                    n534 = local write "操作规范"("顶升油缸已就位，请引进新标准节！" ("字符串")) -> ()
                    n535 = local write "new picture"(w979) -> ()
                  }
                }
                n536 = case shown="真" w916 {
                  frame False {
                    n537 = call "Empty Picture"() -> ("empty picture"=w970:picture)
                    n538 = local write "new picture"(w970) -> ()
                    n539 = local write "操作规范"("" ("字符串")) -> ()
                  }
                  frame True {
                    n540 = call <vilib>:"Read PNG File.vi"("path to PNG file"=path "Picture_Data/1.png" ("path to JPEG file")) -> ("image data"=w976:T2)  [unwired: 8 in, 2 out]
                    n541 = call <vilib>:"Draw Flattened Pixmap.vi"("image data"=w976) -> ("new picture"=w972:picture)  [unwired: 8 in]
                    n542 = One Button Dialog(message="新标准节已引进，请压缩油缸！" ("消息")) -> ()  [unwired: 1 in, 1 out]
                    n543 = local write "操作规范"("新标准节已引进，请压缩油缸！" ("字符串")) -> ()
                    n544 = local write "new picture"(w972) -> ()
                  }
                }
              }
              frame 170..180 {
                n545 = One Button Dialog(message="顶升冒顶警告！" ("消息")) -> ()  [unwired: 1 in, 1 out]
              }
              frame 110..115 {
                n546 = Equal?(x=w997, y=1) -> (x = y?=w1024:bool)
                n547 = Equal?(x=w996, y=1) -> (x = y?=w1025:bool)
                n548 = Equal?(x=w986, y=0) -> (x = y?=w1035:bool)
                n549 = Equal?(x=w985, y=1) -> (x = y?=w1036:bool)
                n550 = Equal?(x=w987, y=0) -> (x = y?=w1034:bool)
                n551 = Equal?(x=w989, y=0) -> (x = y?=w1032:bool)
                n552 = Equal?(x=w995, y=0) -> (x = y?=w1026:bool)
                n553 = Equal?(x=w990, y=0) -> (x = y?=w1031:bool)
                n554 = Equal?(x=w992, y=0) -> (x = y?=w1029:bool)
                n555 = Equal?(x=w993, y=0) -> (x = y?=w1028:bool)
                n556 = Equal?(x=w991, y=0) -> (x = y?=w1030:bool)
                n557 = Equal?(x=w988, y=0) -> (x = y?=w1033:bool)
                n558 = Equal?(x=w994, y=0) -> (x = y?=w1027:bool)
                n559 = Compound Arithmetic op=AND ("复合运算")(w1024, w1025, w1026, w1027, w1028, w1029, w1030, w1031, w1032, w1033, w1034, w1035, w1036) -> (w1050:bool)
                n560 = Equal?(x=w997, y=1) -> (x = y?=w1049:bool)
                n561 = Equal?(x=w996, y=1) -> (x = y?=w1048:bool)
                n562 = Equal?(x=w986, y=1) -> (x = y?=w1038:bool)
                n563 = Equal?(x=w985, y=1) -> (x = y?=w1037:bool)
                n564 = Equal?(x=w987, y=1) -> (x = y?=w1039:bool)
                n565 = Equal?(x=w989, y=1) -> (x = y?=w1041:bool)
                n566 = Equal?(x=w995, y=0) -> (x = y?=w1047:bool)
                n567 = Equal?(x=w990, y=0) -> (x = y?=w1042:bool)
                n568 = Equal?(x=w992, y=0) -> (x = y?=w1044:bool)
                n569 = Equal?(x=w993, y=0) -> (x = y?=w1045:bool)
                n570 = Equal?(x=w991, y=0) -> (x = y?=w1043:bool)
                n571 = Equal?(x=w988, y=1) -> (x = y?=w1040:bool)
                n572 = Equal?(x=w994, y=0) -> (x = y?=w1046:bool)
                n573 = Compound Arithmetic op=AND ("复合运算")(w1049, w1048, w1047, w1046, w1045, w1044, w1043, w1042, w1041, w1040, w1039, w1038, w1037) -> (w1051:bool)
                n574 = case shown="真" w1051 {
                  frame False {
                    n575 = call "Empty Picture"() -> ("empty picture"=w1052:picture)
                    n576 = local write "new picture"(w1052) -> ()
                    n577 = local write "操作规范"("" ("字符串")) -> ()
                  }
                  frame True {
                    n578 = call <vilib>:"Read PNG File.vi"("path to PNG file"=path "Picture_Data/1.png" ("path to JPEG file")) -> ("image data"=w1058:T2)  [unwired: 8 in, 2 out]
                    n579 = call <vilib>:"Draw Flattened Pixmap.vi"("image data"=w1058) -> ("new picture"=w1054:picture)  [unwired: 8 in]
                    n580 = One Button Dialog(message="标准节与塔身已连接，请压缩油缸！" ("消息")) -> ()  [unwired: 1 in, 1 out]
                    n581 = local write "new picture"(w1054) -> ()
                    n582 = local write "操作规范"("标准节与塔身已连接，请压缩油缸！" ("字符串")) -> ()
                  }
                }
                n583 = case shown="真" w1050 {
                  frame False {
                    n584 = call "Empty Picture"() -> ("empty picture"=w1059:picture)
                    n585 = local write "new picture"(w1059) -> ()
                    n586 = local write "操作规范"("" ("字符串")) -> ()
                  }
                  frame True {
                    n587 = call <vilib>:"Read PNG File.vi"("path to PNG file"=path "Picture_Data/1.png" ("path to JPEG file")) -> ("image data"=w1065:T2)  [unwired: 8 in, 2 out]
                    n588 = call <vilib>:"Draw Flattened Pixmap.vi"("image data"=w1065) -> ("new picture"=w1061:picture)  [unwired: 8 in]
                    n589 = One Button Dialog(message="油缸已就位，请连接引进节与塔身！" ("消息")) -> ()  [unwired: 1 in, 1 out]
                    n590 = local write "new picture"(w1061) -> ()
                    n591 = local write "操作规范"("油缸已就位，请连接引进节与塔身！" ("字符串")) -> ()
                  }
                }
              }
            }
            "data out" <- w391
          }
        }
        n592 = property on="数据输出" class="Str"("Text.Scroll Position"=inf) -> ()  [unwired: 2 in, 2 out]
      }
    }
    n593 = case shown="假" "清空" {
      frame False {
      }
      frame True {
        n594 = local write "数据输出"("" ("数据输出")) -> ()
      }
    }
    n595 = call <vilib>:"Read PNG File.vi"("path to PNG file"=path "Picture_Data/jacking_beam.png" ("path to JPEG file")) -> ("image data"=w26:T2)  [unwired: 8 in, 2 out]
    n596 = call <vilib>:"Read PNG File.vi"("path to PNG file"=path "Picture_Data/rotary_support.png" ("path to JPEG file")) -> ("image data"=w15:T2)  [unwired: 8 in, 2 out]
    n597 = call <vilib>:"Read PNG File.vi"("path to PNG file"=path "Picture_Data/pin_shaft.png" ("path to JPEG file")) -> ("image data"=w21:T2)  [unwired: 8 in, 2 out]
    n598 = call <vilib>:"Read PNG File.vi"("path to PNG file"=path "Picture_Data/section_connect.png" ("path to JPEG file")) -> ("image data"=w12:T2)  [unwired: 8 in, 2 out]
    n599 = call <vilib>:"Draw Flattened Pixmap.vi"("image data"=w26) -> ("new picture"=→"jacking_beam":picture)  [unwired: 8 in]
    n600 = call <vilib>:"Read PNG File.vi"("path to PNG file"=path "Picture_Data/stanard_section.png" ("path to JPEG file")) -> ("image data"=w20:T2)  [unwired: 8 in, 2 out]
    n601 = call <vilib>:"Draw Flattened Pixmap.vi"("image data"=w15) -> ("new picture"=→"rotary_support":picture)  [unwired: 8 in]
    n602 = call <vilib>:"Draw Flattened Pixmap.vi"("image data"=w21) -> ("new picture"=→"pin_shaft":picture)  [unwired: 8 in]
    n603 = call <vilib>:"Draw Flattened Pixmap.vi"("image data"=w12) -> ("new picture"=→"section_connect":picture)  [unwired: 8 in]
    n604 = call <vilib>:"Draw Flattened Pixmap.vi"("image data"=w20) -> ("new picture"=→"stanard_section":picture)  [unwired: 8 in]
  }
  n605 = UDP Close(connection ID=w2, 8:w3) -> ()  [unwired: 2 out]
